vi "Post-Install Custom Action.vi"(10 "Variant":variant) -> (0 "error out":errorcluster)   [LabVIEW 2014]
panel:
  # "DCAF requires a few open-source tools to operate.\n\nYou'll be prompted to install these now.  If you do not install these tools, portions of \nDCAF may not work correctly."
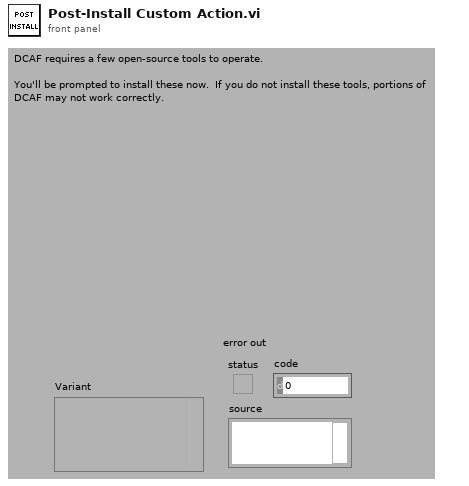
[diagram p1: front panel]
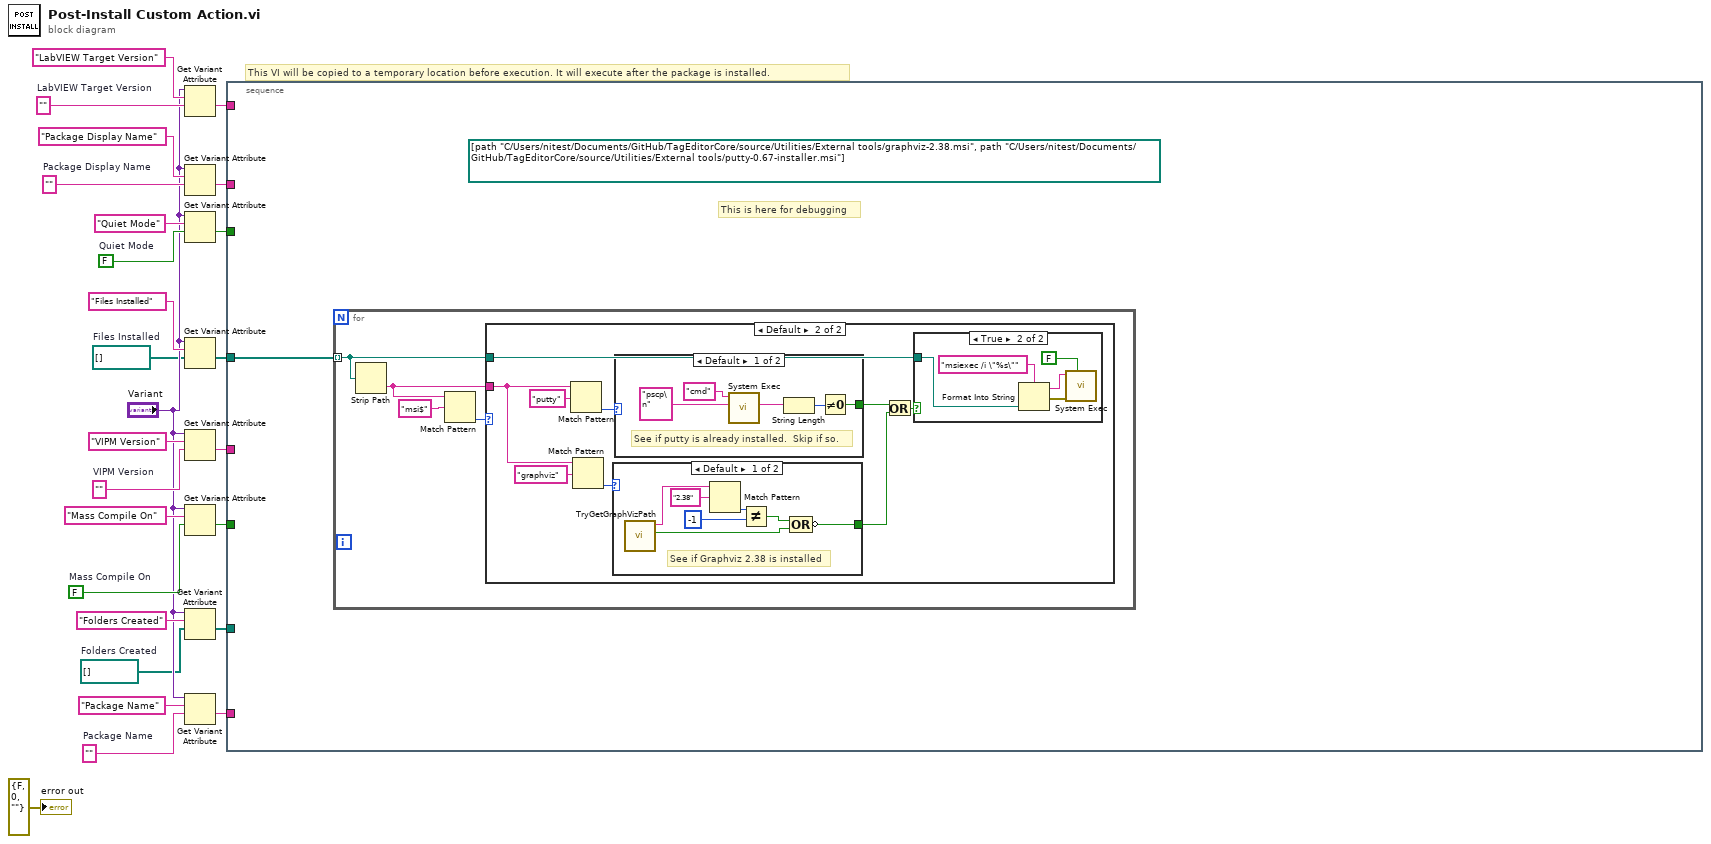
[diagram p0: block diagram]
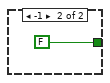
[diagram p3: hidden frame]
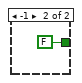
[diagram p5: hidden frame]
diagram:
  w1 = path[] []  # Folders Created
  w2 = path[] []  # Files Installed
  w8 = FALSE  # Mass Compile On
  w9 = ""  # Package Display Name
  w16 = FALSE  # Quiet Mode
  w19 = ""  # VIPM Version
  w21 = ""  # LabVIEW Target Version
  w23 = ""  # Package Name
  # "This VI will be copied to a temporary location before execution. It will execute after the package is installed."
  n1 = Get Variant Attribute(Variant="Variant", name="LabVIEW Target Version", default value (empty Variant)=w21) -> (value=w13:string)  [unwired: 1 in, 3 out]
  n2 = Get Variant Attribute(Variant="Variant", name="Package Display Name", default value (empty Variant)=w9) -> (value=w15:string)  [unwired: 1 in, 3 out]
  n3 = Get Variant Attribute(Variant="Variant", name="Quiet Mode", default value (empty Variant)=w16) -> (value=w11:bool)  [unwired: 1 in, 3 out]
  n4 = Get Variant Attribute(Variant="Variant", name="Files Installed", default value (empty Variant)=w2) -> (value=w5:path[])  [unwired: 1 in, 3 out]
  n5 = Get Variant Attribute(Variant="Variant", name="VIPM Version", default value (empty Variant)=w19) -> (value=w12:string)  [unwired: 1 in, 3 out]
  n6 = Get Variant Attribute(Variant="Variant", name="Mass Compile On", default value (empty Variant)=w8) -> (value=w10:bool)  [unwired: 1 in, 3 out]
  n7 = Get Variant Attribute(Variant="Variant", name="Folders Created", default value (empty Variant)=w1) -> (value=w6:path[])  [unwired: 1 in, 3 out]
  n8 = Get Variant Attribute(Variant="Variant", name="Package Name", default value (empty Variant)=w23) -> (value=w14:string)  [unwired: 1 in, 3 out]
  n9 = stacked-sequence {
    tunnel: w15 -> [_]
    tunnel: w14 -> [_]
    tunnel: w13 -> [_]
    tunnel: w12 -> [_]
    tunnel: w11 -> [_]
    tunnel: w10 -> [_]
    tunnel: w5 -> [w27]
    tunnel: w6 -> [_]
    frame #0 {
      (unwired) path[] [path "C:/Users/nitest/Documents/GitHub/TagEditorCore/source/Utilities/External tools/graphviz-2.38.msi", path "C:/Users/nitest/Documents/GitHub/TagEditorCore/source/Utilities/External tools/putty-0.67-installer.msi"] ("Files Installed")
      # "This is here for debugging"
      n10 = for {
        tunnel: w27 -> [w29] mode=indexing
        n11 = Strip Path(path=w29) -> (name=w28:string)  [unwired: 1 out]
        n12 = Match Pattern(string=w28, regular expression="msi$") -> (offset past match=w30:i32)  [unwired: 1 in, 3 out]
        n13 = case shown="Default" w30 {
          tunnel: w29 -> [_ w38]
          tunnel: w28 -> [_ w33]
          frame -1 {
          }
          frame Default {
            n14 = Match Pattern(string=w33, regular expression="putty") -> (offset past match=w39:i32)  [unwired: 1 in, 3 out]
            n15 = Match Pattern(string=w33, regular expression="graphviz") -> (offset past match=w36:i32)  [unwired: 1 in, 3 out]
            n16 = case shown="Default" w36 {
              tunnel: [w47 FALSE] -> w32
              frame Default {
                # "See if Graphviz 2.38 is installed"
                n17 = call "TryGetGraphVizPath.vi"() -> ("Found?"=w46:bool, "Path"=w43:string)  [unwired: 10 in]
                n18 = Match Pattern(string=w43, regular expression="2.38") -> (offset past match=w45:i32)  [unwired: 1 in, 3 out]
                n19 = Not Equal?(x=w45, y=-1) -> (x != y?=w41:bool)
                n20 = Compound Arithmetic op=OR(w41, w46) -> (invert w47:bool)
              }
              frame -1 {
              }
            }
            n21 = case shown="Default" w39 {
              tunnel: [w54 FALSE] -> w34
              frame Default {
                # "See if putty is already installed.  Skip if so."
                n22 = call <vilib>:"System Exec.vi"("standard input"="pscp\n", "command line"="cmd") -> ("standard error"=w56:string)  [unwired: 6 in, 3 out]
                n23 = String Length(string=w56) -> (length=w55:i32)
                n24 = Not Equal To 0?(x=w55) -> (x != 0?=w54:bool)
              }
              frame -1 {
              }
            }
            n25 = Or(x=w34, y=w32) -> (x .or. y?=w35:bool)
            n26 = case shown="True" w35 {
              tunnel: w38 -> [_ w50]
              frame False {
              }
              frame True {
                n27 = Format Into String(format string="msiexec /i \"%s\"", w50) -> (resulting string=w51:string, error out=w52:errorcluster)  [unwired: 2 in]
                n28 = call <vilib>:"System Exec.vi"("wait until completion? (T)"=FALSE, "error in (no error)"=w52, "command line"=w51) -> ()  [unwired: 5 in, 4 out]
              }
            }
          }
        }
      }
    }
  }
  "error out" <- errorcluster {"status"=FALSE, "code"=0, "source"=""} ("error out")
